vi "Test for Disable.vi"   [LabVIEW 2014, in "Data Manipulation.lvlib"]
uses:
  Data Manipulation.lvlib
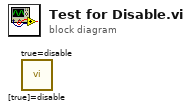
[diagram p0: block diagram]
diagram:
  n1 = call "[true]=disable.vi"() -> ()  [unwired: 3 in, 1 out]
  n2 = call "true=disable.vi"() -> ()  [unwired: 3 in, 1 out]
